vi "Main_v4.vi"() -> ()   [LabVIEW 2018]
uses:
  Clusters/FileDataChannel.ctl
  <vilib>/Platform/TimedLoop/XDataNode/timing_clust.ctl
  <vilib>/Platform/TimedLoop/XDataNode/nitl_modes.ctl
  <vilib>/Platform/TimedLoop/XDataNode/wakeup.ctl
  <vilib>/Analysis/Matrix/Datatypes/RealMatrix.ctl
  Clusters/ArrayPairs.ctl
  Clusters/SwapArrayCluster.ctl
  Clusters/RoscoParams.ctl
  Clusters/SwapIndexes.ctl
  Clusters/SimulationConstants.ctl
  <vilib>/Utility/file.llb/Read Delimited Spreadsheet (DBL).vi
  <vilib>/platform/TimedLoop/XDataNode/XDataNode.xnode
  <vilib>/Platform/TimedLoop/XDataNode/XDNodeRunTimeDep.lvlib
  <vilib>/Analysis/Matrix/NI_Matrix.lvlib
panel:
  out "Iteration Duration":i64
  out "Generator Speed (rad/s)":dbl(slide)=7.068579725455493e-05 scale=-4.0..4.0
  in  "?":T1(tab)
  out "Generator Speed":dbl(graph)
  out "Torque Setpoint (Nm)":sgl(graph)
  out "Pitch Setpoint":sgl(graph)
  in  "To VS_ControlMode":T2(ring)
  in  "Edit DISCON":bool
  out "DISCON.IN Contents":string
  in  "From VS_ControlMode":T2(ring)
  out "avrSWAP":sgl[](array[numeric])
  out "Velocity":dbl
  out "Position":dbl
  out "Cp":dbl[][](array[numeric])
  out "OUT_AERODYN_TQ.Value":sgl
  out "Rotor Speed (rad/s)":sgl(slide)=7.06858e-05 scale=-4.0..4.0
  out "Torque Setpoint (kNm)":sgl(knob) scale=0.0..21586451.0
  out "Pitch Setpoint":sgl(knob) scale=0.0..1.5
  out "Power (kW)":sgl(slide) scale=-15000.0..15000000.0 scale format="%.2f"
  in  "Init WindSpeed(m/s)":sgl=7.0
  in  "File path":path=path "/home/lvuser/rosco-tests"
  out "SimLoop Late?":bool
  out "FIFO Loop Late?":bool
  in  "Base filename":string="rosco-tests"
  out "Writing to cRIO?":bool
  in  "WriteData":bool
  in  "?":T3
  out "#RT FIFO":u32
  out "Call to Rosco Failed?":bool
  out "Rosco Return Message":string
  in  "?":bool
  out "time(s)":dbl
  out "RT Loop Late?":bool
  # "FOCAL Realtime Control (IEA 15MW)"
  # "SENSOR INPUTS"
  # "FILEWRITING SETTINGS"
  # "ERRORS"
  # "TURBINE SPECIFICATIONS"
  # "ROSCO OUTPUTS"
  # "RATED POWER: 15000000 W"
  # "RATED TORQUE: 19624046.66 Nm"
  # "RATED GEN SPEED: 0.79168 rad/s"
  # "ROSCO INPUTS"
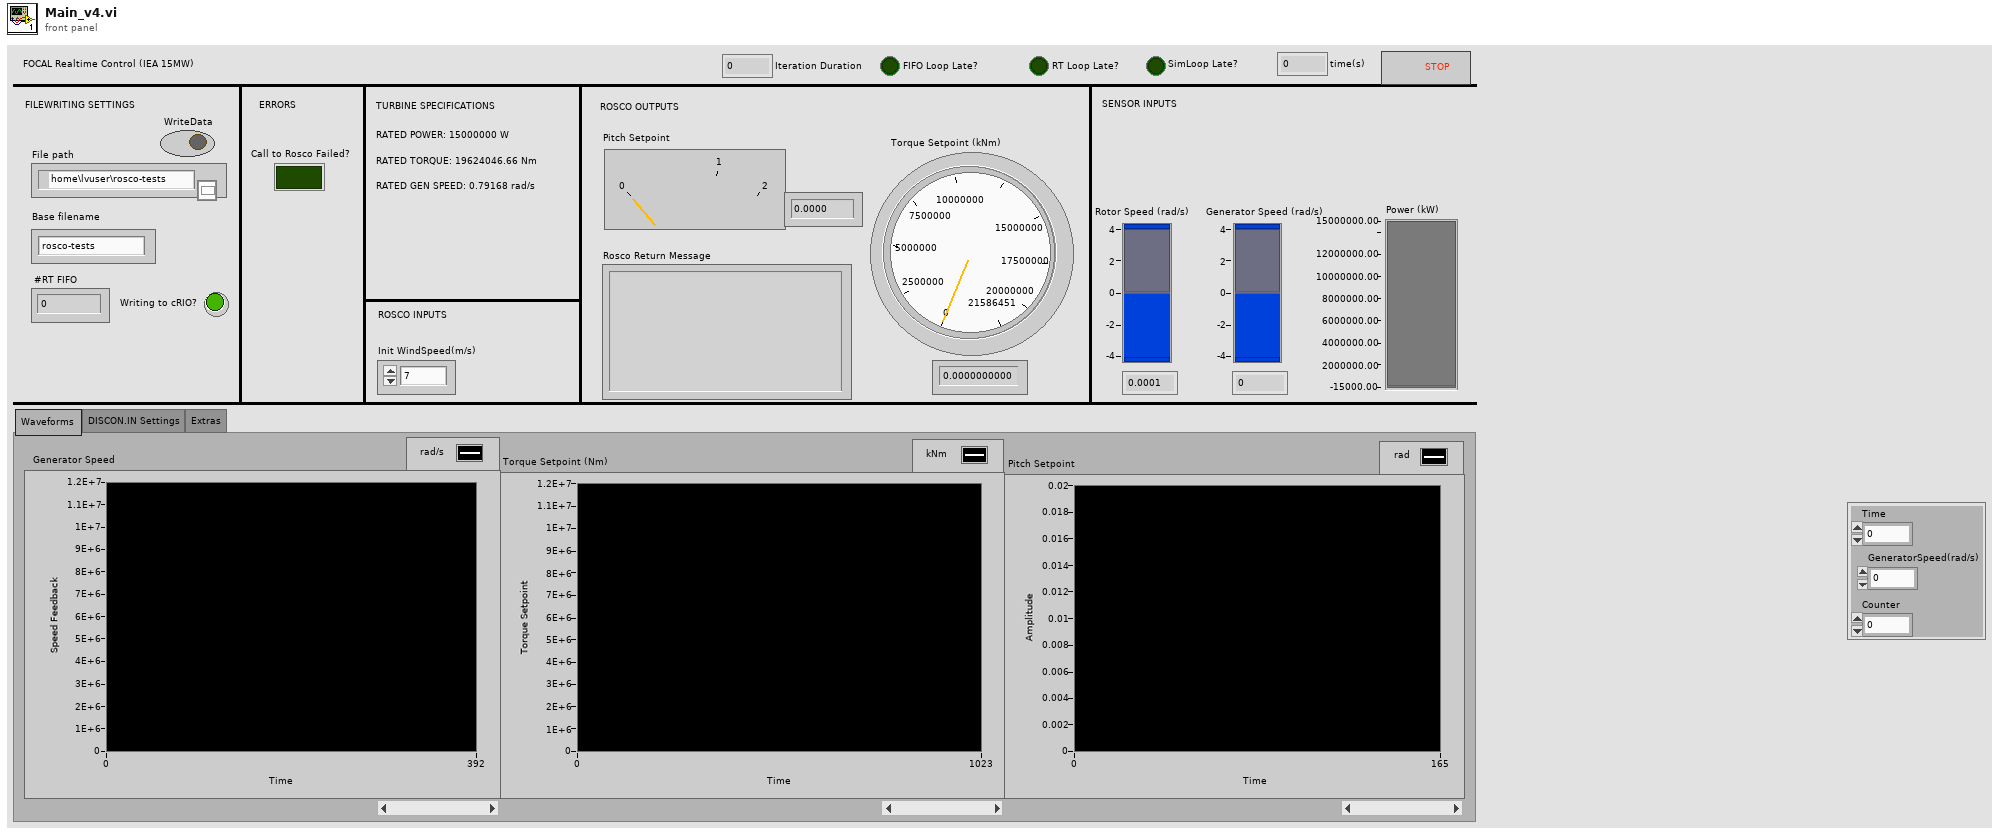
[diagram p1: front panel]
types:
  T1 = enum32{"Waveforms", "DISCON.IN Settings", "Extras"}
  T2 = enum16{"Constant Torque", "Constant Power", "PI Control"}
  T3 = typedef "FileDataChannel.ctl" = cluster{"GeneratorSpeed(rad/s)":sgl, "Counter":sgl, "Time":sgl}
  T4 = typedef "NI_Matrix.lvlib/RealMatrix.ctl" = dbl[][]
  T5 = typedef "ArrayPairs.ctl" = cluster{"iStatus":T6, "TIME":T6, "DT":T6, "BL_PITCH":T6, "VS_MECHGENPWR":T6, "VS_GENPWR":T6, "GEN_SPEED":T6, "ROTOR_SPEED":T6, "GENTQMEAS":T6, "Y_M":T6, "HORWINDV":T6, "ROOTMOOP1":T6, "ROOTMOOP2":T6, "BL_PITCH2":T6, "BL_PITCH3":T6, "ROOTMOOP3":T6, "AVCMSG_SIZE":T6, "INFILE_SIZE ":T6, "OUTFILE_SIZE ":T6, "FA_ACC":T6, "NUM_BLADES":T6, "OUT_BL_PITCH":T6, "OUT_TORQUE":T6, "OUT_AERODYN_TQ":T6}
  T6 = typedef "SwapArrayCluster.ctl" = cluster{"Index":i32, "Value":sgl}
  T7 = typedef "SwapIndexes.ctl" = cluster{"iSTATUS":i32, "TIME":i32, "DT":i32, "BL_PITCH_1":i32, "VS_MECHGENPWR":i32, "GEN_SPEED":i32, "ROT_SPEED":i32, "GENTQMEAS":i32, "Y_M":i32, "HORWINDV":i32, "ROOTMOOP1":i32, "ROOTMOOP2":i32, "BL_PITCH_2":i32, "BL_PITCH_3":i32, "ROOTMOOP3":i32, "INFILE_SIZE":i32, "FA_ACC":i32, "NUM_BLADES":i32, " OUT BL_PITCH":i32, "OUT_ TORQUE":i32, "OUTFILE_SIZE ":i32, "AVCMSG_SIZE":i32, "AERODYN TQ":i32, "VS_GENPWR":i32}
  T8 = typedef "RoscoParams.ctl" = cluster{"avrSWAP":sgl[], "aviFAIL":i32, "avcMSG":string, "ReturnValue":i32}
  T9 = typedef "XDNodeRunTimeDep.lvlib/timing_clust.ctl" = cluster{"Expected End [f-1]":u64, "Actual End [f-1]":u64, "Finished Late? [f-1]":bool, "Expected End [i-1]":u64, "Actual End [i-1]":u64, "Finished Late? [i-1]":bool, "Expected Start [i]":u64, "Actual Start [i]":u64, "Expected Start [f]":u64, "Actual Start [f]":u64, "Source Name":string, "Structure Name":string, "Period":i64, "Deadline":i64, "Offset":i64, "Start":i64, "Priority":i32, "Timeout":i32, "Mode":T10, "Wakeup Reason":T11, "Error":errorcluster, "Source Type":string, "Secondary Source Type":string, "Global End Time":u64, "Global Start Time":u64, "Frame Duration":u64, "Iteration Duration":u64, "Assigned CPU":i32, "I/O Scan Engine Mode":u32}
  T10 = typedef "XDNodeRunTimeDep.lvlib/nitl_modes.ctl" = enum32{"No Change", "Process missed periods, maintain original phase", "Discard missed periods, maintain original phase", "Process missed periods, ignore original phase", "Discard missed periods, ignore original phase"}
  T11 = typedef "XDNodeRunTimeDep.lvlib/wakeup.ctl" = enum32{"Normal", "Aborted", "Asynchronous wakeup", "Timing source error", "Timed loop error", "Timeout"}
  T12 = typedef "SimulationConstants.ctl" = cluster{"Ngear":sgl, "RotorInertia":sgl, "GeneratorEff":sgl, "RotorRadius":sgl, "Rho":sgl}
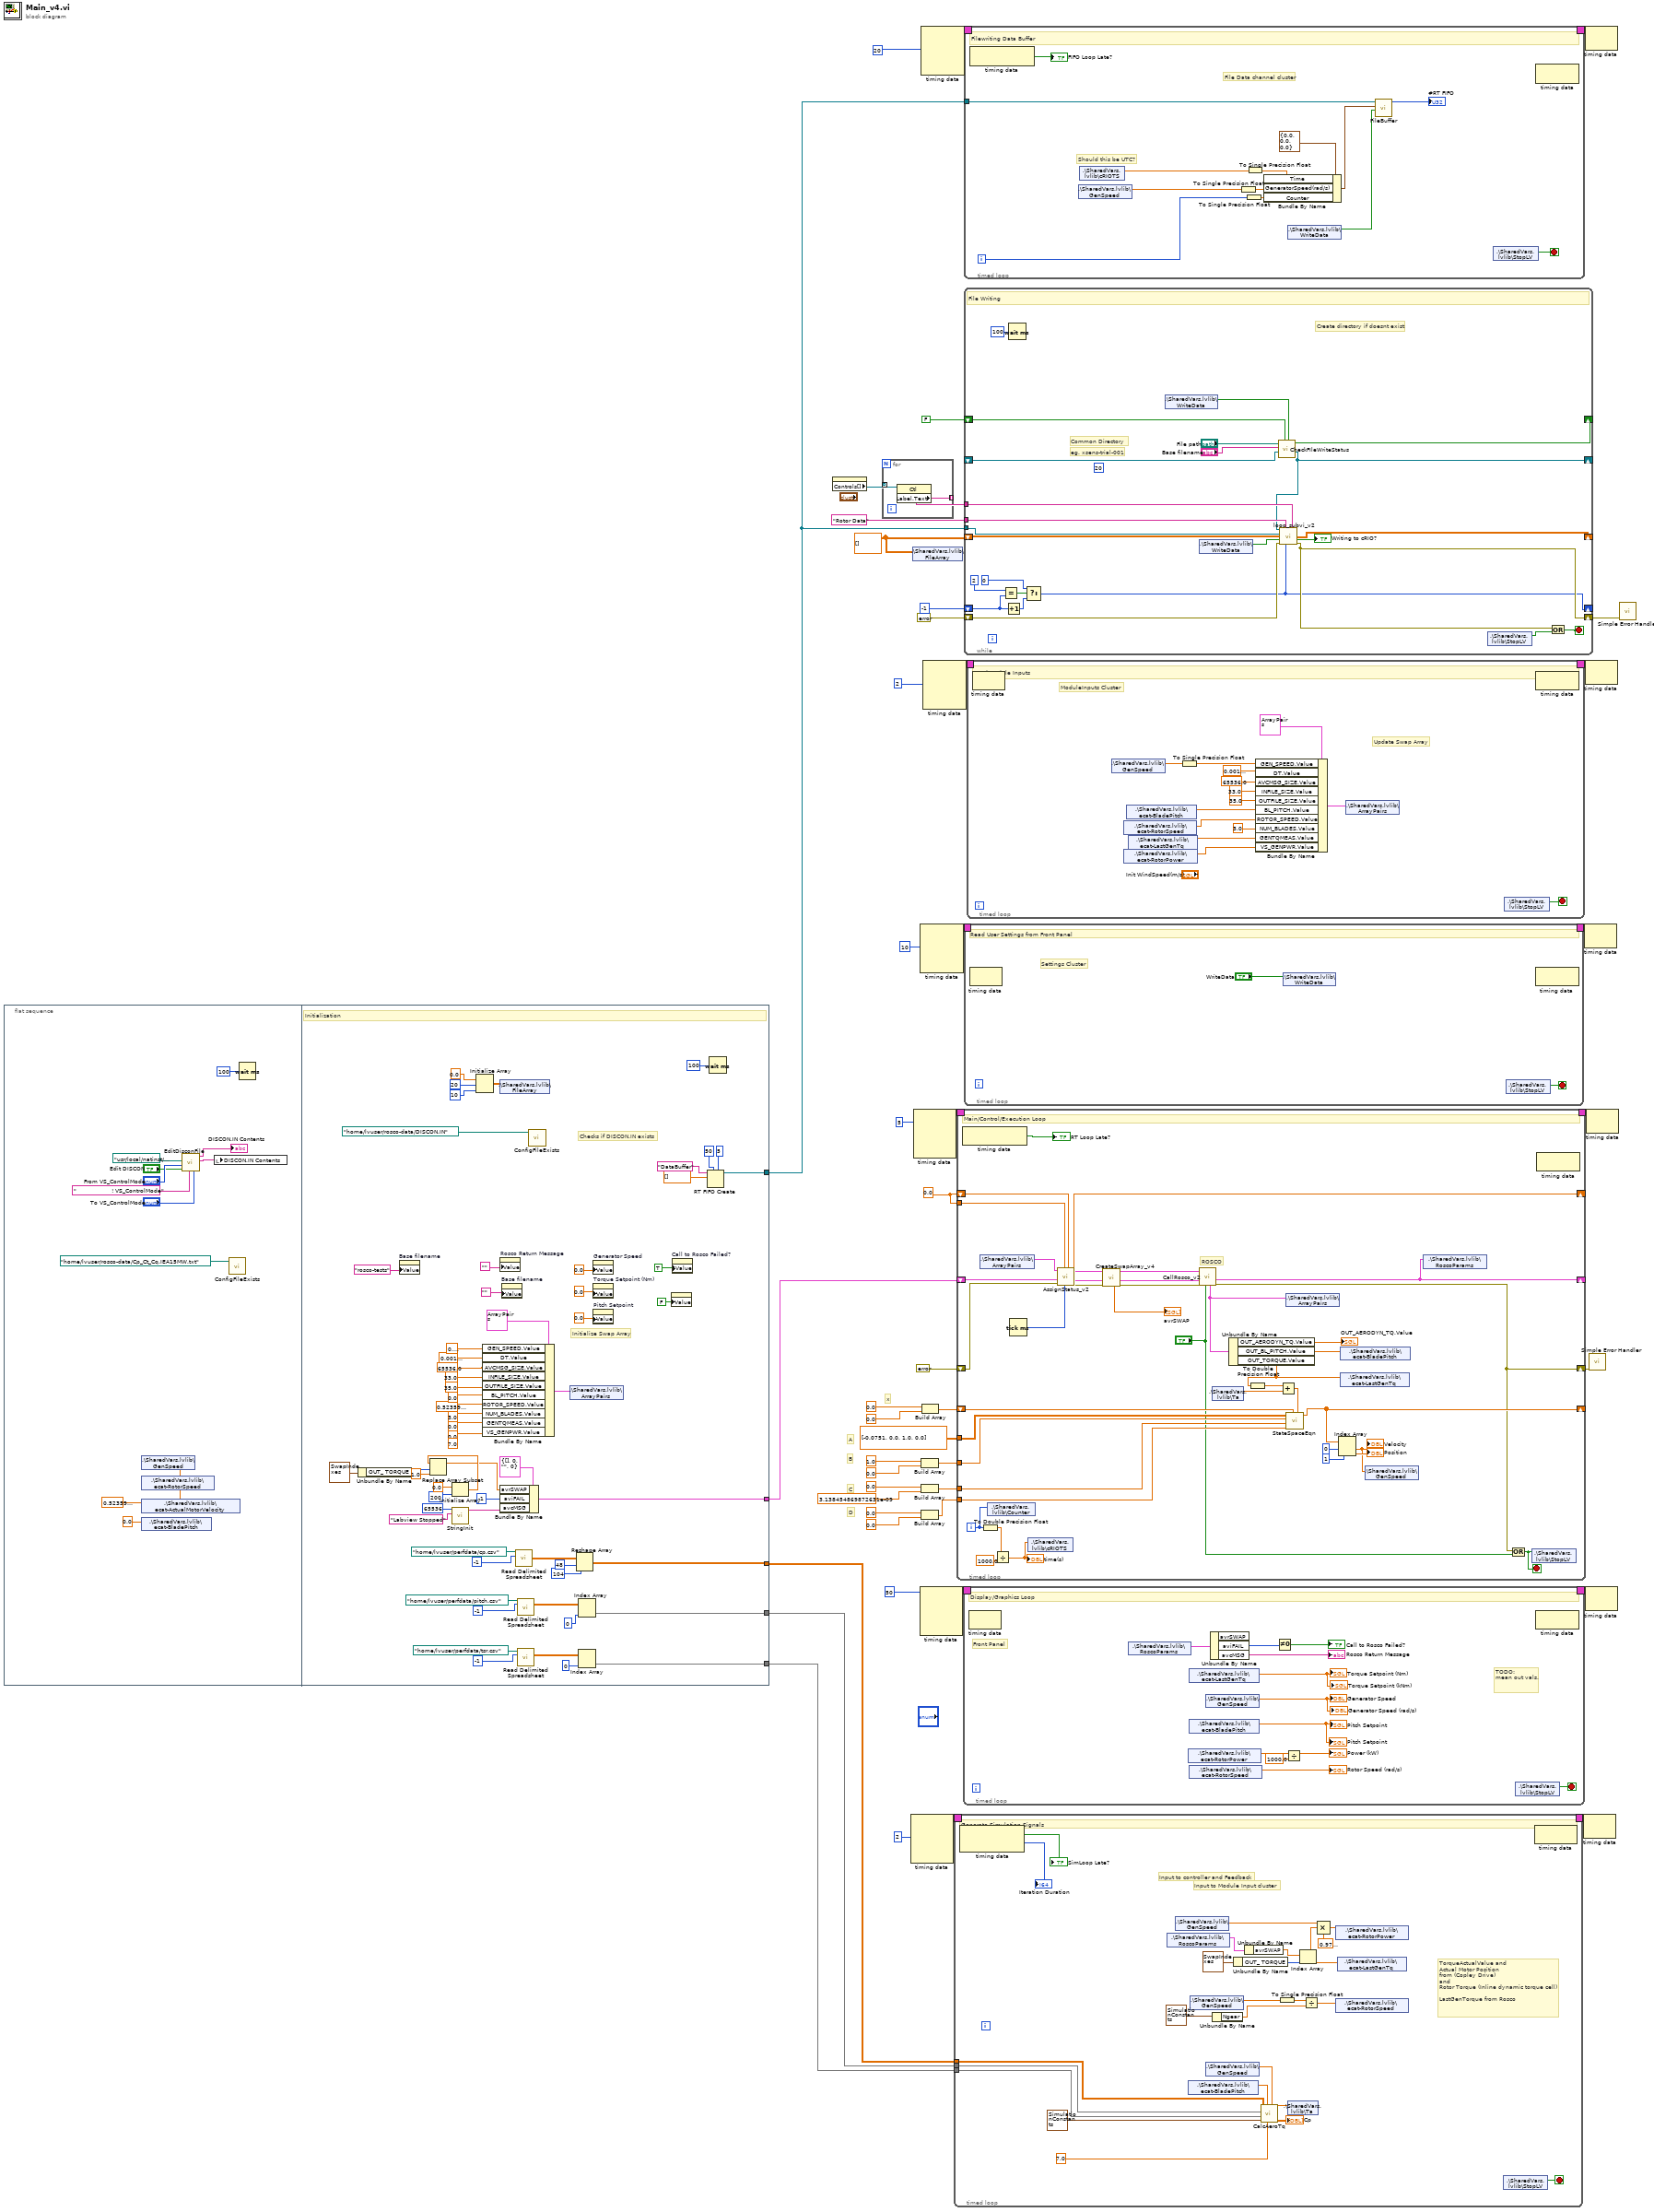
[diagram p0: block diagram]
diagram:
  w24 = dbl[][] [] ("File array 2")
  w31 = 0.0 ("y")
  (unwired) i64 20 ("Period")
  # "A"
  # "B"
  # "D"
  # "C"
  # "x"
  n1 = flat-sequence {
    tunnel: [w109] -> w25
    tunnel: [w94] -> w17
    tunnel: [w83] -> w16
    tunnel: [w78] -> w15
    tunnel: [w77] -> w14
    frame #0 {
      w48 = sgl 0.5236 ("RotorSpeed(rad/s)")
      n2 = shared-variable ".\\SharedVars.lvlib\\GenSpeed"(w48) -> ()  [unwired: 1 in, 1 out]
      n3 = shared-variable ".\\SharedVars.lvlib\\ecat-RotorSpeed"(w48) -> ()  [unwired: 1 in, 1 out]
      n4 = shared-variable ".\\SharedVars.lvlib\\ecat-ActualMotorVelocity"(w48) -> ()  [unwired: 1 in, 1 out]
      n5 = shared-variable ".\\SharedVars.lvlib\\ecat-BladePitch"(sgl 0.0 ("ecat-BladePitch")) -> ()  [unwired: 1 in, 1 out]
      n6 = call "EditDisconFile.vi"("To VS_ControlMode"="To VS_ControlMode", "Append"="                   ! VS_ControlMode", "Edit DISCON"="Edit DISCON", "From VS_ControlMode"="From VS_ControlMode", "path"=path "/usr/local/natinst/labview/DISCON.IN") -> ("result string"=w52:string, "data"=→"DISCON.IN Contents":string)  [unwired: 4 in]
      n7 = local write "DISCON.IN Contents"(w52) -> ()
      n8 = call "ConfigFileExists.vi"("path"=path "/home/lvuser/rosco-data/Cp_Ct_Cq.IEA15MW.txt") -> ()  [unwired: 11 in]
      n9 = Wait (ms)(milliseconds to wait=u32 100) -> ()  [unwired: 1 out]
    }
    frame #1 {
      (unwired) sgl 7.0 ("WindSpeed(m/s)")
      # "Initialize Swap Array"
      # "Checks if DISCON.IN exists"
      # "Initialization"
      n10 = Unbundle By Name(T7 {"iSTATUS"=0, "TIME"=1, "DT"=2, "BL_PITCH_1"=3, "VS_MECHGENPWR"=13, "GEN_SPEED"=19, "ROT_SPEED"=20, "GENTQMEAS"=22, "Y_M"=23, "HORWINDV"=26, "ROOTMOOP1"=29, "ROOTMOOP2"=30, "BL_PITCH_2"=32, "BL_PITCH_3"=33, "ROOTMOOP3"=31, "INFILE_SIZE"=49, "FA_ACC"=52, "NUM_BLADES"=60, " OUT BL_PITCH"=44, "OUT_ TORQUE"=46, "OUTFILE_SIZE "=50, "AVCMSG_SIZE"=48, "AERODYN TQ"=89, "VS_GENPWR"=14} ("Index In")) -> ("OUT_ TORQUE"=w74:i32)
      n11 = property on="Base filename" class="Str"("Value"="rosco-tests" ("Base filename")) -> ()  [unwired: 2 in, 2 out]
      n12 = Initialize Array(sgl 0.0 ("element"), 200 ("dimension size")) -> (w72:sgl[])
      n13 = Replace Array Subset(array=w72, new element=1.0 ("new element/subarray"), index=w74) -> (w71:sgl[])
      n14 = call "StringInit.vi"("accOUTNAME"="Labview Stopped", "dimension size"=65536) -> ("result string"=w113:string)  [unwired: 9 in]
      n15 = Initialize Array(0.0 ("element"), 20 ("dimension size"), 10 ("dimension size")) -> (w105:dbl[][])
      n16 = Bundle By Name(cluster=T5 {"iStatus"={"Index"=0, "Value"=0.0}, "TIME"={"Index"=1, "Value"=0.0}, "DT"={"Index"=2, "Value"=0.0}, "BL_PITCH"={"Index"=3, "Value"=0.0}, "VS_MECHGENPWR"={"Index"=13, "Value"=0.0}, "VS_GENPWR"={"Index"=14, "Value"=0.0}, "GEN_SPEED"={"Index"=19, "Value"=0.0}, "ROTOR_SPEED"={"Index"=20, "Value"=0.0}, "GENTQMEAS"={"Index"=22, "Value"=0.0}, "Y_M"={"Index"=23, "Value"=0.0}, "HORWINDV"={"Index"=26, "Value"=0.0}, "ROOTMOOP1"={"Index"=29, "Value"=0.0}, "ROOTMOOP2"={"Index"=30, "Value"=0.0}, "BL_PITCH2"={"Index"=32, "Value"=0.0}, "BL_PITCH3"={"Index"=33, "Value"=0.0}, "ROOTMOOP3"={"Index"=31, "Value"=0.0}, "AVCMSG_SIZE"={"Index"=48, "Value"=0.0}, "INFILE_SIZE "={"Index"=49, "Value"=0.0}, "OUTFILE_SIZE "={"Index"=50, "Value"=0.0}, "FA_ACC"={"Index"=52, "Value"=0.0}, "NUM_BLADES"={"Index"=60, "Value"=0.0}, "OUT_BL_PITCH"={"Index"=44, "Value"=0.0}, "OUT_TORQUE"={"Index"=46, "Value"=0.0}, "OUT_AERODYN_TQ"={"Index"=89, "Value"=0.0}} ("ArrayPairs"), "GEN_SPEED.Value"=sgl 0.3 ("GeneratorSpeed(rad/s)"), "DT.Value"=sgl 0.001 ("Dt"), "AVCMSG_SIZE.Value"=sgl 65536.0 ("new element/subarray"), "INFILE_SIZE.Value"=sgl 33.0 ("new element/subarray"), "OUTFILE_SIZE.Value"=sgl 35.0 ("new element/subarray"), "BL_PITCH.Value"=sgl 0.0 ("GeneratorTorque(Nm)"), "ROTOR_SPEED.Value"=sgl 0.5236 ("RotorSpeed(rad/s)"), "NUM_BLADES.Value"=sgl 3.0 ("NumberofBlades"), "GENTQMEAS.Value"=sgl 0.0 ("BladePitch(rad)"), "VS_GENPWR.Value"=sgl 0.0 ("Generator Power(W)")) -> (w59:T5)
      n17 = shared-variable ".\\SharedVars.lvlib\\FileArray"(w105) -> ()  [unwired: 1 in, 1 out]
      n18 = Bundle By Name(cluster=T8 {"avrSWAP"=[], "aviFAIL"=0, "avcMSG"="", "ReturnValue"=0}, "avrSWAP"=w71, "aviFAIL"=-1, "avcMSG"=w113) -> (w94:T8)
      n19 = property on="Rosco Return Message" class="Str"("Value"="") -> ()  [unwired: 2 in, 2 out]
      n20 = property on="Base filename" class="Str"("Value"="") -> ()  [unwired: 2 in, 2 out]
      n21 = call-poly <vilib>:"Read Delimited Spreadsheet.vi"("file path (dialog if empty)"=path "/home/lvuser/perfdata/cp.csv", "number of rows (all:-1)"=-1) -> ("all rows"=w86:dbl[][])  [unwired: 8 in, 5 out]
      n22 = call-poly <vilib>:"Read Delimited Spreadsheet.vi"("file path (dialog if empty)"=path "/home/lvuser/perfdata/pitch.csv", "number of rows (all:-1)"=-1) -> ("all rows"=w82:dbl[][])  [unwired: 8 in, 5 out]
      n23 = call-poly <vilib>:"Read Delimited Spreadsheet.vi"("file path (dialog if empty)"=path "/home/lvuser/perfdata/tsr.csv", "number of rows (all:-1)"=-1) -> ("all rows"=w88:dbl[][])  [unwired: 8 in, 5 out]
      n24 = call "ConfigFileExists.vi"("path"=path "/home/lvuser/rosco-data/DISCON.IN") -> ()  [unwired: 11 in]
      n25 = shared-variable ".\\SharedVars.lvlib\\ArrayPairs"(w59) -> ()  [unwired: 1 in, 1 out]
      n26 = Reshape Array(w86, 48 ("dimension size"), 104 ("dimension size")) -> (w83:dbl[][])
      n27 = Index Array(array=w82, index (col)=0 ("disabled index (col)")) -> (element=w78:dbl[])  [unwired: 1 in]
      n28 = Index Array(array=w88, index (col)=0 ("disabled index (col)")) -> (element=w77:dbl[])  [unwired: 1 in]
      n29 = property on="Generator Speed" class="WFChart (strict)"("Value"=sgl 0.0 ("Generator Speed")) -> ()  [unwired: 2 in, 2 out]
      n30 = property on="Torque Setpoint (Nm)" class="WFChart (strict)"("Value"=sgl 0.0 ("Generator Speed")) -> ()  [unwired: 2 in, 2 out]
      n31 = property on="Pitch Setpoint" class="WFChart (strict)"("Value"=sgl 0.0 ("Generator Speed")) -> ()  [unwired: 2 in, 2 out]
      n32 = property class="Bool (strict)"("Value"=FALSE) -> ()  [unwired: 2 in, 2 out]
      n33 = property on="Call to Rosco Failed?" class="Bool (strict)"("Value"=TRUE ("Call to Rosco Failed?")) -> ()  [unwired: 2 in, 2 out]
      n34 = RT FIFO Create(0:"DataBuffer" ("name (unnamed)"), 1:dbl[] [] ("appended array"), 4:u32 50, 6:u32 5) -> (8:w109:refnum<k33>)  [unwired: 4 in, 2 out]
      n35 = Wait (ms)(milliseconds to wait=u32 100) -> ()  [unwired: 1 out]
    }
  }
  n36 = property class="Clust (strict)"() -> ("Controls[]"=w28:refnum<vi>[])  [unwired: 2 in, 2 out]
  n37 = for {
    tunnel: w28 -> [w120] mode=indexing
    tunnel: [w119] -> w27 mode=indexing
    n38 = property class="Ctl"(reference=w120) -> ("Label.Text"=w119:string)  [unwired: 1 in, 2 out]
  }
  n39 = node-c288(i64 2 ("Period")) -> (w39:T9)  [unwired: 3 in]
  n40 = shared-variable ".\\SharedVars.lvlib\\FileArray"(w24) -> ()  [unwired: 1 in, 1 out]
  n41 = node-c288(i64 5 ("Period")) -> (w37:T9)  [unwired: 3 in]
  n42 = node-c288(i64 50 ("Period")) -> (w41:T9)  [unwired: 3 in]
  n43 = node-c288(i64 10 ("Period")) -> (w43:T9)  [unwired: 3 in]
  n44 = node-c288(i64 20 ("Period")) -> (w47:T9)  [unwired: 3 in]
  n45 = Build Array(1.0 ("element"), 0.0 ("element")) -> (w3:dbl[])
  n46 = Build Array(0.0 ("element"), 3.138454869872631e-09 ("element")) -> (w2:dbl[])
  n47 = Build Array(0.0 ("element"), 0.0 ("element")) -> (w1:dbl[])
  n48 = Build Array(0.0 ("element"), 0.0 ("element")) -> (w9:dbl[])
  n49 = node-c288(i64 2 ("Period")) -> (w45:T9)  [unwired: 3 in]
  n50 = timed-loop {
    timing: w39 -> [_]
    timing-out: [_] -> w38
    tunnel: w16 -> [w127]
    tunnel: w15 -> [w126]
    tunnel: w14 -> [w125]
    stop <- w145 stop-if-true
    # "TorqueActualValue and \nActual Motor Position \nfrom (Copley Drive)\nand\nRotor Torque (Inline dynamic torque cell)\n\nLastGenTorque from Rosco"
    # "Input to Module Input cluster"
    # "Input to controller and Feedback"
    # "Generate Simulation Signals"
    n51 = node-c288() -> (→"SimLoop Late?":bool, →"Iteration Duration":i64)  [unwired: 1 in]
    n52 = shared-variable ".\\SharedVars.lvlib\\RoscoParams"() -> (w138:T8)  [unwired: 1 in, 1 out]
    n53 = shared-variable ".\\SharedVars.lvlib\\GenSpeed"() -> (w139:dbl)  [unwired: 1 in, 1 out]
    n54 = shared-variable ".\\SharedVars.lvlib\\ecat-BladePitch"() -> (w129:sgl)  [unwired: 1 in, 1 out]
    n55 = shared-variable ".\\SharedVars.lvlib\\GenSpeed"() -> (w133:dbl)  [unwired: 1 in, 1 out]
    n56 = shared-variable ".\\SharedVars.lvlib\\GenSpeed"() -> (w128:dbl)  [unwired: 1 in, 1 out]
    n57 = Unbundle By Name(T12 {"Ngear"=1.0, "RotorInertia"=318628130.0, "GeneratorEff"=0.97, "RotorRadius"=0.97, "Rho"=0.97} ("SimulationConst")) -> ("Ngear"=w135:sgl)
    n58 = Unbundle By Name(T7 {"iSTATUS"=0, "TIME"=1, "DT"=2, "BL_PITCH_1"=3, "VS_MECHGENPWR"=13, "GEN_SPEED"=19, "ROT_SPEED"=20, "GENTQMEAS"=22, "Y_M"=23, "HORWINDV"=26, "ROOTMOOP1"=29, "ROOTMOOP2"=30, "BL_PITCH_2"=32, "BL_PITCH_3"=33, "ROOTMOOP3"=31, "INFILE_SIZE"=49, "FA_ACC"=52, "NUM_BLADES"=60, " OUT BL_PITCH"=44, "OUT_ TORQUE"=46, "OUTFILE_SIZE "=50, "AVCMSG_SIZE"=48, "AERODYN TQ"=89, "VS_GENPWR"=14} ("Index In")) -> ("OUT_ TORQUE"=w140:i32)
    n59 = Unbundle By Name(w138) -> ("avrSWAP"=w141:sgl[])
    n60 = call "CalcAeroTq.vi"("GenSpeed"=w128, "WindSpeed"=sgl 7.0, "Xi"=w129, "SimulationConst"=T12 {"Ngear"=1.0, "RotorInertia"=318628130.0, "GeneratorEff"=0.97, "RotorRadius"=0.97, "Rho"=0.97}, "tsr(Y)"=w125, "pitch (X)"=w126, "Cp(Z)"=w127) -> ("Cp"=→"Cp":dbl[][], "Ta"=w121:dbl)  [unwired: 3 in]
    n61 = To Single Precision Float(number=w133) -> (single precision float=w132:sgl)
    n62 = shared-variable ".\\SharedVars.lvlib\\Ta"(w121) -> ()  [unwired: 1 in, 1 out]
    n63 = Index Array(array=w141, index=w140) -> (element=w144:sgl)
    n64 = Divide(x=w132, y=w135) -> (x/y=w134:sgl)
    n65 = Compound Arithmetic op=MULTIPLY(w139, w144, sgl 0.97 ("value")) -> (w142:dbl)
    n66 = shared-variable ".\\SharedVars.lvlib\\ecat-RotorPower"(w142) -> ()  [unwired: 1 in, 1 out]
    n67 = shared-variable ".\\SharedVars.lvlib\\ecat-RotorSpeed"(w134) -> ()  [unwired: 1 in, 1 out]
    n68 = shared-variable ".\\SharedVars.lvlib\\ecat-LastGenTq"(w144) -> ()  [unwired: 1 in, 1 out]
    n69 = shared-variable ".\\SharedVars.lvlib\\StopLV"() -> (w145:bool)  [unwired: 1 in, 1 out]
    n70 = node-c288() -> ()  [unwired: 1 in, 1 out]
  }
  n71 = timed-loop {
    timing: w37 -> [_]
    timing-out: [_] -> w36
    shift-right: [w165] -> _
    shift-left: w31 -> [w167]
    tunnel: w31 -> [w166]
    shift-right: [w156] -> _
    shift-left: w17 -> [w170]
    shift-right: [w157] -> w18
    shift-left: errorcluster {"status"=FALSE, "code"=0, "source"=""} ("error out") -> [w169]
    shift-right: [w179] -> _
    shift-left: w9 -> [w184]
    tunnel: T4 [[-0.0751, 0.0], [1.0, 0.0]] ("A") -> [w183]
    tunnel: w3 -> [w182]
    tunnel: w2 -> [w181]
    tunnel: w1 -> [w180]
    i -> [w185]
    stop <- w186 stop-if-true
    # "ROSCO"
    # "Main/Control/Execution Loop"
    n72 = node-c288() -> (→"RT Loop Late?":bool)  [unwired: 1 in]
    n73 = shared-variable ".\\SharedVars.lvlib\\ArrayPairs"() -> (w171:T5)  [unwired: 1 in, 1 out]
    n74 = To Double Precision Float(number=w185) -> (double precision float=w188:dbl)
    n75 = shared-variable ".\\SharedVars.lvlib\\Counter"(w185) -> ()  [unwired: 1 in, 1 out]
    n76 = Divide(x=w188, y=1000.0) -> (x/y=w150:dbl)
    "time(s)" <- w150
    n77 = Tick Count (ms)() -> (millisecond timer value=w168:u32)
    n78 = shared-variable ".\\SharedVars.lvlib\\cRIOTS"(w150) -> ()  [unwired: 1 in, 1 out]
    n79 = call "AssignStatus_v2.vi"("LoopCount"=w167, "Time"=w168, "Init Val"=w166, "error in (no error)"=w169, "ROSCO Params"=w170, "ArrayPairs In"=w171) -> ("error out"=w162:errorcluster, "ROSCO Params 2"=w163:T8, "ArrayPairs Out"=w164:T5, "Count+1"=w165:dbl)  [unwired: 2 in]
    n80 = call "CreateSwapArray_v4.vi"("error in (no error)"=w162, "ROSCO Params"=w163, "ArrayPairs"=w164) -> ("error out"=w158:errorcluster, "ROSCO Params Out"=w159:T8, "ArrayPairs Out"=w160:T5, "avrSWAP"=→"avrSWAP":sgl[])  [unwired: 5 in]
    n81 = call "CallRosco_v2.vi"("StopLV"="?", "error in (no error)"=w158, "ROSCO Params in"=w159, "ArrayPairs"=w160) -> ("error out"=w157:errorcluster, "ROSCO Params out"=w156:T8, "ArrayPairs 2"=w153:T5)  [unwired: 5 in]
    n82 = shared-variable ".\\SharedVars.lvlib\\Ta"() -> (w173:dbl)  [unwired: 1 in, 1 out]
    n83 = Unbundle By Name(w153) -> ("OUT_AERODYN_TQ.Value"=→"OUT_AERODYN_TQ.Value":sgl, "OUT_BL_PITCH.Value"=w154:sgl, "OUT_TORQUE.Value"=w152:sgl)
    n84 = To Double Precision Float(number=w152) -> (double precision float=w174:dbl)
    n85 = Add(x=w174, y=w173) -> (x+y=w172:dbl)
    n86 = shared-variable ".\\SharedVars.lvlib\\ArrayPairs"(w153) -> ()  [unwired: 1 in, 1 out]
    n87 = call "StateSpaceEqn.vi"("u"=w172, "x"=w184, "D"=w180, "C"=w181, "B"=w182, "A"=w183) -> ("x(t+1)"=w179:dbl[])  [unwired: 4 in, 1 out]
    n88 = Index Array(array=w179, index #1=0 ("index"), index #2=1 ("index")) -> (element #1=w175:dbl, element #2=→"Position":dbl)
    "Velocity" <- w175
    n89 = shared-variable ".\\SharedVars.lvlib\\ecat-BladePitch"(w154) -> ()  [unwired: 1 in, 1 out]
    n90 = shared-variable ".\\SharedVars.lvlib\\ecat-LastGenTq"(w152) -> ()  [unwired: 1 in, 1 out]
    n91 = shared-variable ".\\SharedVars.lvlib\\GenSpeed"(w175) -> ()  [unwired: 1 in, 1 out]
    n92 = shared-variable ".\\SharedVars.lvlib\\RoscoParams"(w156) -> ()  [unwired: 1 in, 1 out]
    n93 = Or(x=w157, y="?") -> (x .or. y?=w186:bool)
    n94 = shared-variable ".\\SharedVars.lvlib\\StopLV"(w186) -> ()  [unwired: 1 in, 1 out]
    n95 = node-c288() -> ()  [unwired: 1 in, 1 out]
  }
  n96 = timed-loop {
    timing: w41 -> [_]
    timing-out: [_] -> w40
    stop <- w204 stop-if-true
    # "TODO:\nmean out vals."
    # "Front Panel"
    # "Display/Graphics Loop"
    n97 = node-c288() -> ()  [unwired: 1 in, 1 out]
    n98 = shared-variable ".\\SharedVars.lvlib\\RoscoParams"() -> (w203:T8)  [unwired: 1 in, 1 out]
    n99 = shared-variable ".\\SharedVars.lvlib\\ecat-RotorPower"() -> (w199:sgl)  [unwired: 1 in, 1 out]
    n100 = shared-variable ".\\SharedVars.lvlib\\ecat-RotorSpeed"() -> (→"Rotor Speed (rad/s)":sgl)  [unwired: 1 in, 1 out]
    n101 = shared-variable ".\\SharedVars.lvlib\\ecat-LastGenTq"() -> (→"Torque Setpoint (Nm)" →"Torque Setpoint (kNm)":sgl)  [unwired: 1 in, 1 out]
    n102 = shared-variable ".\\SharedVars.lvlib\\ecat-BladePitch"() -> (→"Pitch Setpoint" →"Pitch Setpoint":sgl)  [unwired: 1 in, 1 out]
    n103 = shared-variable ".\\SharedVars.lvlib\\GenSpeed"() -> (→"Generator Speed" →"Generator Speed (rad/s)":dbl)  [unwired: 1 in, 1 out]
    n104 = Unbundle By Name(w203) -> ("aviFAIL"=w201:i32, "avcMSG"=→"Rosco Return Message":string)  [unwired: 1 out]
    n105 = Not Equal To 0?(x=w201) -> (x != 0?=→"Call to Rosco Failed?":bool)
    n106 = Divide(x=w199, y=sgl 1000.0) -> (x/y=→"Power (kW)":sgl)
    n107 = shared-variable ".\\SharedVars.lvlib\\StopLV"() -> (w204:bool)  [unwired: 1 in, 1 out]
    n108 = node-c288() -> ()  [unwired: 1 in, 1 out]
  }
  n109 = while {
    shift-right: [w207] -> _
    shift-left: _ -> [w208]
    shift-right: [w215] -> _
    shift-left: FALSE -> [w216]
    shift-right: [w228] -> w20
    shift-left: errorcluster {"status"=FALSE, "code"=0, "source"=""} ("error out") -> [w227]
    tunnel: "Rotor Data" -> [w210]
    tunnel: w27 -> [w211]
    tunnel: w25 -> [w212]
    shift-right: [w224] -> _
    shift-left: -1 -> [w226]
    shift-right: [w219] -> _
    shift-left: w24 -> [w225]
    stop <- w230 stop-if-true
    # "eg. xsens-trial-001"
    # "Create directory if doesnt exist"
    # "Common Directory"
    # "File Writing"
    n110 = Equal?(x=2 ("t"), y=w226) -> (x = y?=w221:bool)
    n111 = Increment(x=w226) -> (x+1=w220:i32)
    n112 = Wait (ms)(milliseconds to wait=u32 100) -> ()  [unwired: 1 out]
    n113 = Select(t=0, s=w221, f=w220) -> (s? t:f=w224:i32)
    n114 = shared-variable ".\\SharedVars.lvlib\\WriteData"() -> (w217:bool)  [unwired: 1 in, 1 out]
    n115 = shared-variable ".\\SharedVars.lvlib\\WriteData"() -> (w213:bool)  [unwired: 1 in, 1 out]
    n116 = call "CheckFIleWriteStatus.vi"("WriteDataButtonVal"=w217, "WritePrevVal"=w216, "Refnum in"=w208, "Base filename"="Base filename", "File path"="File path") -> ("Refnum out"=w207:refnum<k34>, "WriteCurrentVal"=w215:bool)  [unwired: 5 in]
    n117 = call "loop_subvi_v2.vi"("Refnum in"=w207, "Group Name"=w210, "Channel Names"=w211, "rt fifo"=w212, "File array"=w225, "Write?"=w213, "error in (no error)"=w227, "index"=w224) -> ("File array 2"=w219:dbl[][], "Writing to file"=→"Writing to cRIO?":bool, "error out"=w228:errorcluster)  [unwired: 4 in, 1 out]
    n118 = shared-variable ".\\SharedVars.lvlib\\StopLV"() -> (w231:bool)  [unwired: 1 in, 1 out]
    n119 = Or(x=w228, y=w231) -> (x .or. y?=w230:bool)
  }
  n120 = timed-loop {
    timing: w43 -> [_]
    timing-out: [_] -> w42
    stop <- w233 stop-if-true
    # "Settings Cluster"
    # "Read User Settings from Front Panel"
    n121 = node-c288() -> ()  [unwired: 1 in, 1 out]
    n122 = shared-variable ".\\SharedVars.lvlib\\WriteData"("WriteData") -> ()  [unwired: 1 in, 1 out]
    n123 = shared-variable ".\\SharedVars.lvlib\\StopLV"() -> (w233:bool)  [unwired: 1 in, 1 out]
    n124 = node-c288() -> ()  [unwired: 1 in, 1 out]
  }
  n125 = timed-loop {
    timing: w47 -> [_]
    timing-out: [_] -> w46
    tunnel: w25 -> [w242]
    i -> [w239]
    stop <- w248 stop-if-true
    # "Should this be UTC?"
    # "File Data channel cluster"
    # "Filewriting Data Buffer"
    n126 = node-c288() -> (→"FIFO Loop Late?":bool)  [unwired: 1 in]
    n127 = shared-variable ".\\SharedVars.lvlib\\GenSpeed"() -> (w247:dbl)  [unwired: 1 in, 1 out]
    n128 = shared-variable ".\\SharedVars.lvlib\\cRIOTS"() -> (w236:dbl)  [unwired: 1 in, 1 out]
    n129 = To Single Precision Float(number=w247) -> (single precision float=w237:sgl)
    n130 = To Single Precision Float(number=w239) -> (single precision float=w240:sgl)
    n131 = To Single Precision Float(number=w236) -> (single precision float=w246:sgl)
    n132 = Bundle By Name(cluster=T3 {"GeneratorSpeed(rad/s)"=0.0, "Counter"=0.0, "Time"=0.0} ("SwapIn"), "Time"=w246, "GeneratorSpeed(rad/s)"=w237, "Counter"=w240) -> (w244:T3)
    n133 = shared-variable ".\\SharedVars.lvlib\\WriteData"() -> (w243:bool)  [unwired: 1 in, 1 out]
    n134 = call "FileBuffer.vi"("Boolean"=w243, "FileDataChannel"=w244, "Refnum in"=w242) -> ("# elements"=→"#RT FIFO":u32)  [unwired: 8 in]
    n135 = shared-variable ".\\SharedVars.lvlib\\StopLV"() -> (w248:bool)  [unwired: 1 in, 1 out]
    n136 = node-c288() -> ()  [unwired: 1 in, 1 out]
  }
  n137 = timed-loop {
    timing: w45 -> [_]
    timing-out: [_] -> w44
    stop <- w265 stop-if-true
    # "Update Swap Array"
    # "ModuleInputs Cluster"
    # "Read Module Inputs"
    n138 = node-c288() -> ()  [unwired: 1 in, 1 out]
    n139 = shared-variable ".\\SharedVars.lvlib\\GenSpeed"() -> (w260:dbl)  [unwired: 1 in, 1 out]
    n140 = shared-variable ".\\SharedVars.lvlib\\ecat-RotorSpeed"() -> (w257:sgl)  [unwired: 1 in, 1 out]
    n141 = shared-variable ".\\SharedVars.lvlib\\ecat-RotorPower"() -> (w254:sgl)  [unwired: 1 in, 1 out]
    n142 = shared-variable ".\\SharedVars.lvlib\\ecat-BladePitch"() -> (w258:sgl)  [unwired: 1 in, 1 out]
    n143 = shared-variable ".\\SharedVars.lvlib\\ecat-LastGenTq"() -> (w255:sgl)  [unwired: 1 in, 1 out]
    n144 = To Single Precision Float(number=w260) -> (single precision float=w259:sgl)
    n145 = Bundle By Name(cluster=T5 {"iStatus"={"Index"=0, "Value"=0.0}, "TIME"={"Index"=1, "Value"=0.0}, "DT"={"Index"=2, "Value"=0.0}, "BL_PITCH"={"Index"=3, "Value"=0.0}, "VS_MECHGENPWR"={"Index"=13, "Value"=0.0}, "VS_GENPWR"={"Index"=14, "Value"=0.0}, "GEN_SPEED"={"Index"=19, "Value"=0.0}, "ROTOR_SPEED"={"Index"=20, "Value"=0.0}, "GENTQMEAS"={"Index"=22, "Value"=0.0}, "Y_M"={"Index"=23, "Value"=0.0}, "HORWINDV"={"Index"=26, "Value"=0.0}, "ROOTMOOP1"={"Index"=29, "Value"=0.0}, "ROOTMOOP2"={"Index"=30, "Value"=0.0}, "BL_PITCH2"={"Index"=32, "Value"=0.0}, "BL_PITCH3"={"Index"=33, "Value"=0.0}, "ROOTMOOP3"={"Index"=31, "Value"=0.0}, "AVCMSG_SIZE"={"Index"=48, "Value"=0.0}, "INFILE_SIZE "={"Index"=49, "Value"=0.0}, "OUTFILE_SIZE "={"Index"=50, "Value"=0.0}, "FA_ACC"={"Index"=52, "Value"=0.0}, "NUM_BLADES"={"Index"=60, "Value"=0.0}, "OUT_BL_PITCH"={"Index"=44, "Value"=0.0}, "OUT_TORQUE"={"Index"=46, "Value"=0.0}, "OUT_AERODYN_TQ"={"Index"=89, "Value"=0.0}} ("ArrayPairs"), "GEN_SPEED.Value"=w259, "DT.Value"=sgl 0.001 ("Dt"), "AVCMSG_SIZE.Value"=sgl 65536.0 ("new element/subarray"), "INFILE_SIZE.Value"=sgl 33.0 ("new element/subarray"), "OUTFILE_SIZE.Value"=sgl 35.0 ("new element/subarray"), "BL_PITCH.Value"=w258, "ROTOR_SPEED.Value"=w257, "NUM_BLADES.Value"=sgl 3.0 ("NumberofBlades"), "GENTQMEAS.Value"=w255, "VS_GENPWR.Value"=w254) -> (w252:T5)
    n146 = shared-variable ".\\SharedVars.lvlib\\ArrayPairs"(w252) -> ()  [unwired: 1 in, 1 out]
    n147 = shared-variable ".\\SharedVars.lvlib\\StopLV"() -> (w265:bool)  [unwired: 1 in, 1 out]
    n148 = node-c288() -> ()  [unwired: 1 in, 1 out]
  }
  n149 = node-c288(w38) -> ()  [unwired: 1 out]
  n150 = node-c288(w42) -> ()  [unwired: 1 out]
  n151 = node-c288(w46) -> ()  [unwired: 1 out]
  n152 = node-c288(w44) -> ()  [unwired: 1 out]
  n153 = node-c288(w40) -> ()  [unwired: 1 out]
  n154 = node-c288(w36) -> ()  [unwired: 1 out]
  n155 = call <vilib>:"Simple Error Handler.vi"("error in (no error)"=w18) -> ()  [unwired: 4 in, 5 out]
  n156 = call <vilib>:"Simple Error Handler.vi"("error in (no error)"=w20) -> ()  [unwired: 4 in, 5 out]
